vi "Read Weight Tool Vacuum.vi"(8 "error in":errorcluster, 11 "Gantry in":refnum<class "Gantry Class.lvclass">) -> (0 "error out":errorcluster, 2 "On/Off":bool, 3 "Gantry out":refnum<class "Gantry Class.lvclass">)   [LabVIEW 2011, in "Gantry Class.lvclass"]
uses:
  Gantry Class.lvclass
  WorkTable Class/WorkTable Class.lvclass
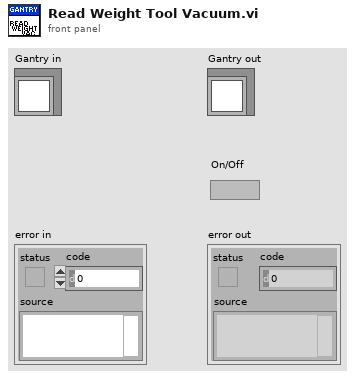
[diagram p1: front panel]
types:
  T1 = typedef "Worktable_Weights.ctl" = cluster{"Weight Slots":T2[], "Vacuum Channel":i32}
  T2 = typedef "Worktable_Weight.ctl" = cluster{"Weight State":enum16{"Empty", "Populated"}, "Weight Type":T3, "Location/Orientation":T4}
  T3 = typedef "Weight Type.ctl" = enum16{"Weight 1", "Weight 2", "Weight 3", "Weight 4", "Weight 5", "Weight 6", "Weight 7", "Weight 8"}
  T4 = typedef "Position_Orientation.ctl" = cluster{"Center":refnum<class "Vec3d Class.lvclass">, "Orientation":refnum<class "Orient3d Class.lvclass">}
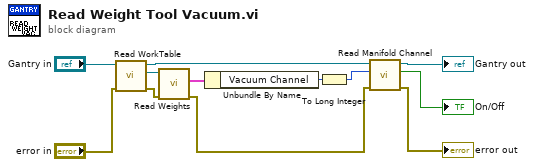
[diagram p0: block diagram]
diagram:
  n1 = call-dynamic "Read WorkTable.vi"("error in"="error in", "Gantry Class in"="Gantry in") -> ("error out"=w4:errorcluster, "WorkTable Class.lvclass"=w6:refnum<class "WorkTable Class.lvclass">, "Gantry Class out"=w7:refnum<class "Gantry Class.lvclass">)  [unwired: 7 in]
  n2 = call-dynamic "Read Weights.vi"("error in (no error)"=w4, "WorkTable Class in"=w6) -> ("error out"=w3:errorcluster, "Weights"=w5:T1)  [unwired: 7 in, 1 out]
  n3 = Unbundle By Name(w5) -> ("Vacuum Channel"=w2:i32)
  n4 = To Long Integer(number=w2) -> (32bit integer=w1:i32)
  n5 = call-dynamic "Read Manifold Channel.vi"("error in"=w3, "Manifold Channel"=w1, "Gantry in"=w7) -> ("error out"=→"error out":errorcluster, "On/Off"=→"On/Off":bool, "Gantry out"=→"Gantry out":refnum<class "Gantry Class.lvclass">)  [unwired: 6 in]
